vi "sound.vi"() -> ()   [LabVIEW 2016]
uses:
  <vilib>/Simulation/Scripting/Companion Diagram/SimConfigNode/SimDog.xnode
  <vilib>/Simulation/Implementation/Shared/SIMSCR Execution Mode.ctl
  <vilib>/Simulation/Scripting/Companion Diagram/SimConfigNode/_simSolvers.ctl
  <vilib>/Simulation/Scripting/Companion Diagram/SimConfigNode/SimParams.ctl
  <vilib>/Simulation/Implementation/XNodeFramework/SimXNode/SimX.xnode
  <vilib>/Simulation/ContinuousLinear/Implementation/NILVSim Integrator new.llb/SIM Integrator (scalar).vi
  <vilib>/Simulation/SignalDisplay/Implementation/NILVSim Time Waveform.llb/SIM Time Waveform (scalar).vi
  <vilib>/Simulation/SignalDisplay/Implementation/NILVSim Buffer XY Graph.llb/SIM Buffer XY Graph (scalar).vi
  <vilib>/Simulation/ContinuousLinear/Implementation/NILVSim Transfer Function Direct.llb/SIM Transfer Function Direct (SISO).vi
  <vilib>/Simulation/SignalArithmetic/Implementation/NILVSim Gain.llb/SIM Gain (scalar).vi
  <vilib>/Simulation/Nonlinear/Implementation/NILVSim Switch.llb/SIM Switch (scalar).vi
  <vilib>/Simulation/Utility/Implementation/SIM Time.vi
  <vilib>/Analysis/baseanly.llb/Histogram.vi
  <vilib>/Analysis/NI_AALBase.lvlib
  <vilib>/gmath/trans.llb/STFT Spectrograms.vi
  <vilib>/gmath/NI_Gmath.lvlib
panel:
  out "Acquired time domain signal 3":waveform(dbl)(graph)={"t0"=timestamp(0 s since 1904-01-01), "dt"=0.001, "Y"=[]}
  out "Acquired time domain signal 2":waveform(dbl)(graph)={"t0"=timestamp(0 s since 1904-01-01), "dt"=0.001, "Y"=[]}
  out "Acquired time domain signal":waveform(dbl)(graph)={"t0"=timestamp(0 s since 1904-01-01), "dt"=0.001, "Y"=[]}
  in  "Frequency bins":i32=512
  in  "Time steps":i32(slide)=2 scale=2.0..20.0
  in  "Length":i32=64
  in  "Type":u32(ring)=1 items=["Rectangle"=0, "Hanning"=1, "Hamming"=2, "Blackman-Harris"=3, "Exact Blackman"=4, "Blackman"=5, "Flat Top"=6, "4 Term B-Harris "=7, "7 Term B-Harris"=8, "Low Sidelobe"=9, "Blackman Nuttall"=11, "Triangle"=30, "Bartlett-Hanning"=31, "Bohman"=32, "Parzen"=33, "Welch"=34, "Kaiser"=60, "Dolph-Chebyshev"=61, "Gaussian"=62]
  in  "Window parameter":dbl=nan
  out "3":dbl[][](graph)
  out "2 2":dbl[][](graph)
  out "2":dbl[][](graph)
  out "histogram":T1(graph)
  out "?":T1(graph)
  out "2":T1(graph)
  out "size(s)":i32
  in  "Sample rate (Hz)":dbl=22050.0
  in  "Duration (s)":dbl=1.0
  out "e3":waveform(dbl)(graph)
  out "e2":waveform(dbl)(graph)
  out "e1":waveform(dbl)(graph)
  out "X m":waveform(dbl)(graph)
  out "Y  m":waveform(dbl)(graph)
  out "YZ m":cluster{dbl, dbl}[](graph)
  out "XY m":cluster{dbl, dbl}[](graph)
  out "XZ m":cluster{dbl, dbl}[](graph)
  out "Z  m":waveform(dbl)(graph)
  out "XYs":cluster{dbl, dbl}[](graph)
  out "XZs":cluster{dbl, dbl}[](graph)
  out "YZs":cluster{dbl, dbl}[](graph)
  out "Zs":waveform(dbl)(graph)
  out "Ys":waveform(dbl)(graph)
  out "Xs":waveform(dbl)(graph)
  # "1234"
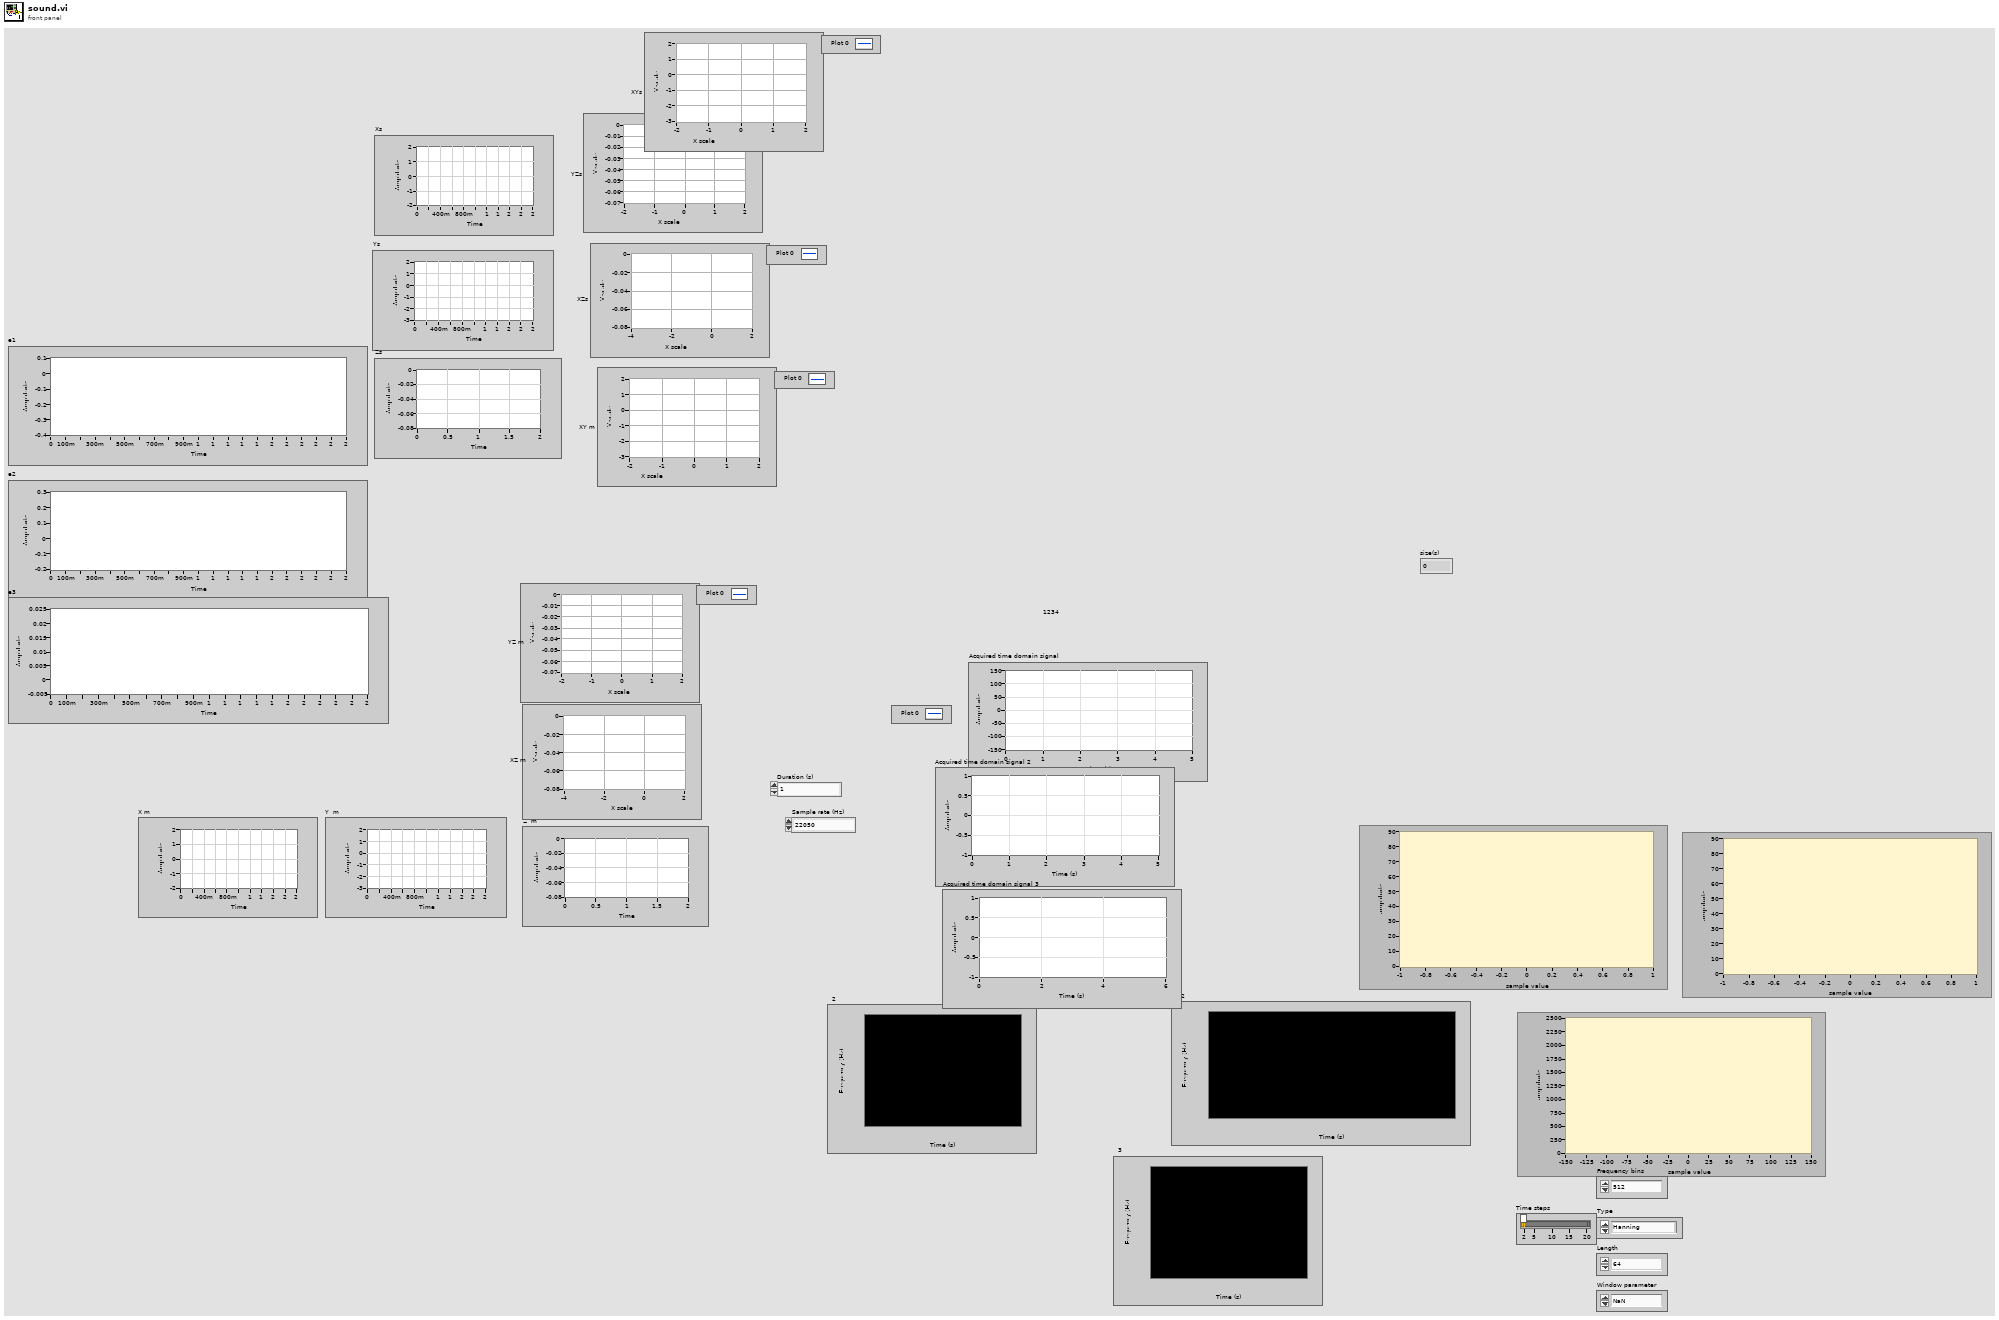
[diagram p1: front panel]
types:
  T1 = cluster{"X Values":dbl[], "Histogram: h(x)":i32[]}
  T2 = typedef "SimParams.ctl" = cluster{"Initial Time (s)":dbl, "Final Time (s)":dbl, "Step Size (s)":dbl, "ODE Solver":T3, "Minimum Step Size (s)":dbl, "Maximum Step Size (s)":dbl, "Relative Tolerance":dbl, "Absolute Tolerance":dbl, "Software Timing":bool, "Initial Step Size (s)":dbl, "Automatic Fixed Step Size?":bool, "Automatic Discrete Step Size?":bool, "Discrete Step Size (s)":dbl, "Calculate using Time Step":bool, "Solver Wired?":bool, "Prev.Frm.Expected End":u64, "Prev.Frm.Actual End":u64, "Prev.Frm.Finished Late?":bool, "Prev.Iter.Expected End":u64, "Prev.Iter.Actual End":u64, "Prev.Iter.Finished Late?":bool, "Expected Iteration Start":u64, "Actual Iteration Start":u64, "Expected Frame Start":u64, "Actual Frame Start":u64, "Source Name":string, "Name":string, "Period":i64, "Deadline":i64, "Offset":i64, "Start":i64, "Priority":i32, "Timeout":i32, "Processor":i32, "Mode":enum32{"No Change", "Process missed periods, maintain original phase", "Discard missed periods, maintain original phase", "Process missed periods, ignore original phase", "Discard missed periods, ignore original phase"}, "Wakeup reason":enum32{"Normal", "Aborted", "Asynchronous wakeup", "Timing source error", "Timed loop error", "Timeout"}, "Error":errorcluster, "Source Type":string, "Secondary Source Type":string, "Global End Time":u64, "Global Start Time":u64, "Full Solver Reset":bool, "Execution Mode":T4, "Nan/Inf Check":bool, "Custom Solver Library":string, "Solver Is Variable":bool, "custom solver name":string, "Signal Collection Decimation":u32}
  T3 = typedef "_simSolvers.ctl" = enum16{"Runge-Kutta 1 (Euler)", "Runge-Kutta 2", "Runge-Kutta 3", "Runge-Kutta 4", "Runge-Kutta 23 (variable)", "Runge-Kutta 45 (variable)", "BDF (variable)", "Adams-Moulton (variable)", "Rosenbrock (variable)", "Discrete States Only", "SDIRK 4 (variable)", "Radau 5 (variable)", "Radau 9 (variable)", "Radau 13 (variable)", "Radau [Variable Order] (variable)", "Gear's Method (variable)", "Linearizer", "State Query", "Trim Eval", "Custom Solver"}
  T4 = typedef "SIMSCR Execution Mode.ctl" = enum16{"Simulate to Completion", "Single Time-Step Simulation (Fixed Step Only)"}
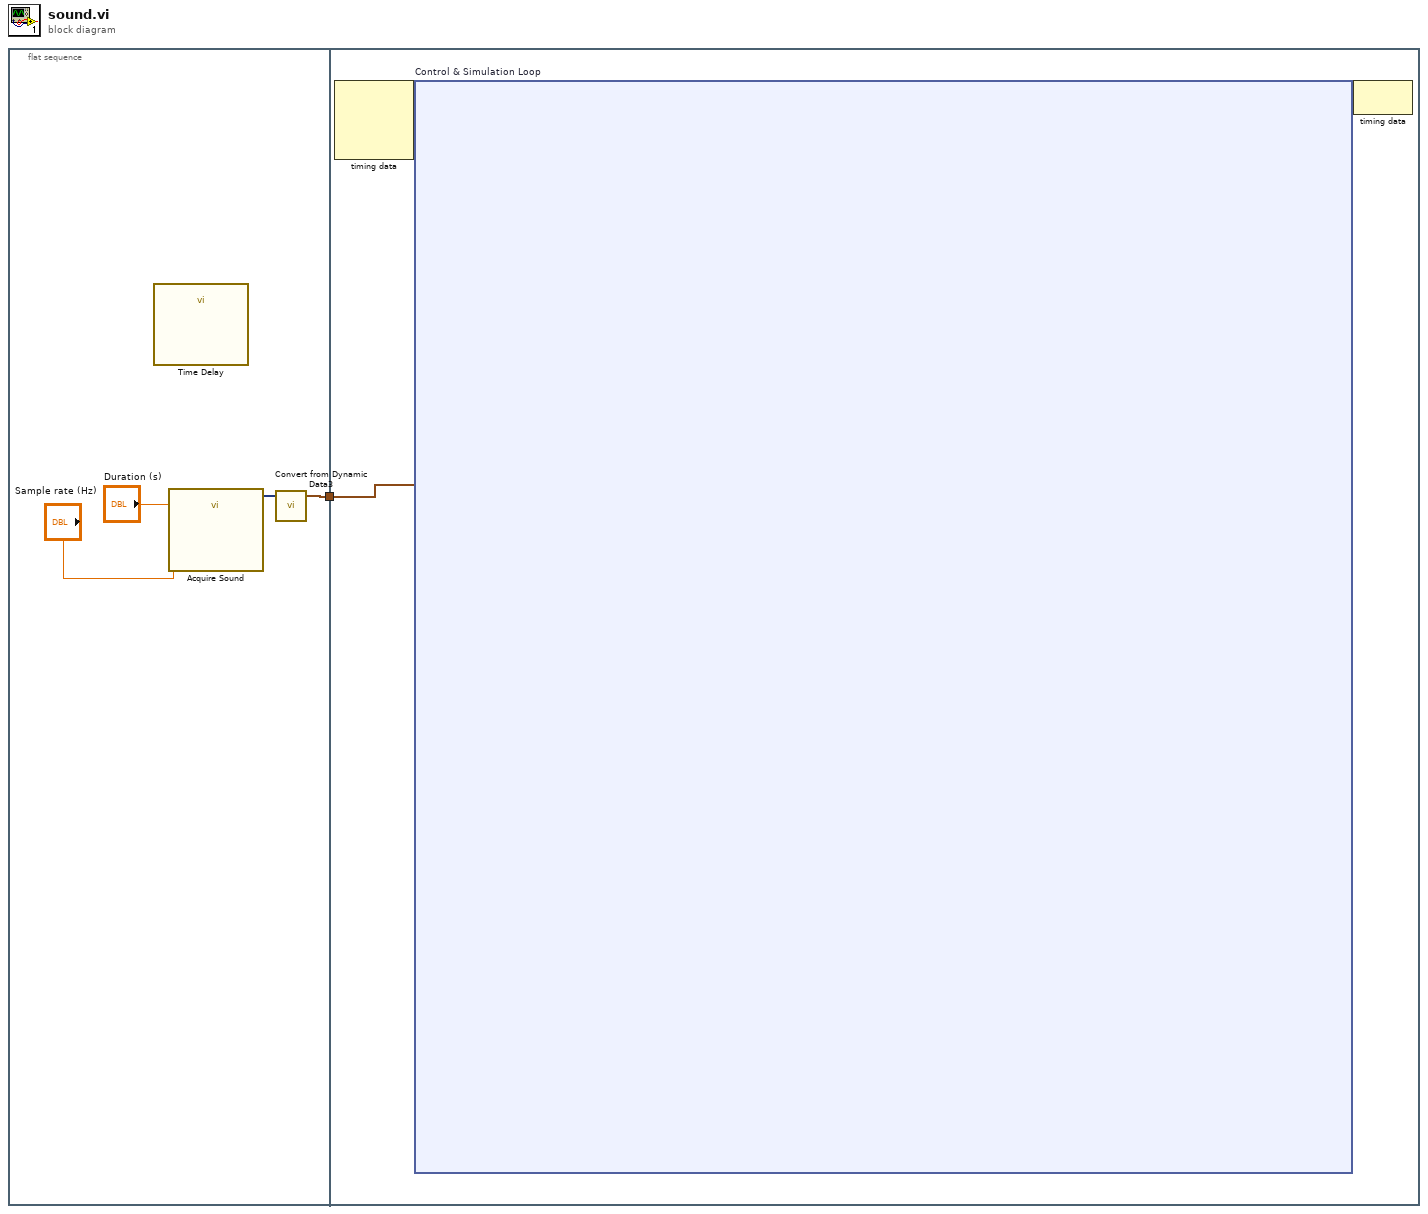
[diagram p0: block diagram]
diagram:
  n1 = flat-sequence {
    tunnel: [w2] -> w1
    tunnel: w1 -> [w6]
    frame #0 {
      n2 = call "Time Delay"() -> ()  [unwired: 11 in, 1 out]
      n3 = call "Acquire Sound"("Duration (s)"="Duration (s)", "Sample rate (Hz)"="Sample rate (Hz)") -> ("Data"=w3:dynamicdata)  [unwired: 16 in, 1 out]
      n4 = call "Convert from Dynamic Data3"("Dynamic Data Type"=w3) -> ("Waveform"=w2:waveform(dbl))  [unwired: 3 in]
    }
    frame #1 {
      n5 = node-c288() -> (w8:variant)  [unwired: 4 in]
      n6 = node-c254 "Control & Simulation Loop"(w8, w6) -> (w7:variant)  [unwired: 1 out]
      n7 = node-c288(w7) -> ()  [unwired: 1 out]
    }
  }
